vi "uc480_SetExposure.vi"(0 ".NET (Reference) In":refnum<k24>, 7 "Exposure time":dbl, 11 "Error In":errorcluster) -> (15 "Error out":errorcluster caption="Error Out")   [LabVIEW 2021]
uses:
  C:/Program Files/Thorlabs/Scientific Imaging/ThorCam/uc480DotNet.dll
  Program Files/Thorlabs/Scientific Imaging/ThorCam/uc480DotNet.dll
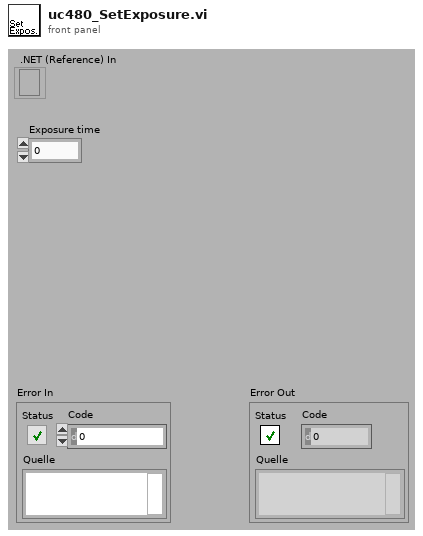
[diagram p1: front panel]
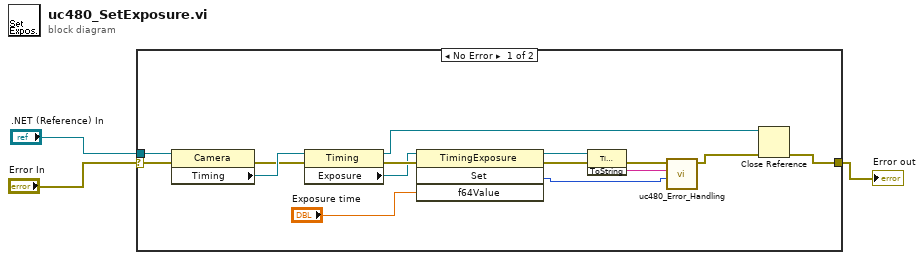
[diagram p0: block diagram]
diagram:
  n1 = case shown="No Error" "Error In" {
    selector: "Error In" -> [w4 w19]
    tunnel: ".NET (Reference) In" -> [w14 _]
    tunnel: [w13 w19] -> w2
    frame No Error {
      n2 = property class="Camera"(reference=w14, error in=w4) -> (error out=w17:errorcluster, "Timing"=w18:refnum<k24>)  [unwired: 1 out]
      n3 = property class="Timing"(reference=w18, error in=w17) -> (reference out=w12:refnum<k24>, error out=w16:errorcluster, "Exposure"=w15:refnum<k24>)
      n4 = invoke class="TimingExposure" method="Set"(reference=w15, error in=w16, "f64Value"="Exposure time") -> (reference out=w10:refnum<k24>, error out=w9:errorcluster, "Set"=w6:i32)  [unwired: 1 in, 1 out]
      n5 = invoke class="TimingExposure" method="ToString"(reference=w10, error in=w9) -> (error out=w8:errorcluster, "ToString"=w7:string)  [unwired: 1 in, 1 out]
      n6 = call "uc480_Error_Handling.vi"("Error Code"=w6, "Error String"=w7, "Error In"=w8) -> ("Error Out"=w5:errorcluster)  [unwired: 8 in]
      n7 = Close Reference(reference=w12, error in (no error)=w5) -> (error out=w13:errorcluster)
    }
    frame Error {
    }
  }
  "Error out" <- w2
